vi "Image to 24bit Pixmap.vi"(8 "Columns":i32, 10 "Rows":i32, 11 "image":u8[](array[numeric])) -> (2 "Array":u32[][](array[numeric]))   [LabVIEW 2020]
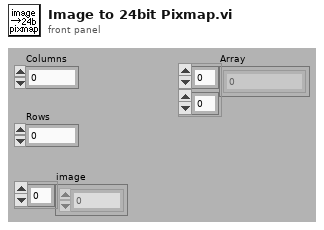
[diagram p1: front panel]
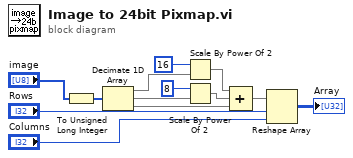
[diagram p0: block diagram]
diagram:
  n1 = To Unsigned Long Integer(number="image") -> (unsigned 32bit integer=w12:u32[])
  n2 = Decimate 1D Array(w12) -> (w4:u32[], w5:u32[], w6:u32[])
  n3 = Scale By Power Of 2(n=i16 16, x=w4) -> (x*2^n=w8:u32[])
  n4 = Scale By Power Of 2(n=i16 8, x=w5) -> (x*2^n=w7:u32[])
  n5 = Compound Arithmetic op=ADD(w8, w7, w6) -> (w9:u32[])
  n6 = Reshape Array(w9, "Rows", "Columns") -> (→"Array":u32[][])
